vi "DumbDash Send.vi"(9 "Robot IP":string, 10 "data string":string) -> ()   [LabVIEW 2015]
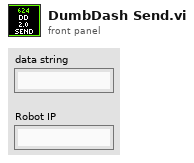
[diagram p1: front panel]
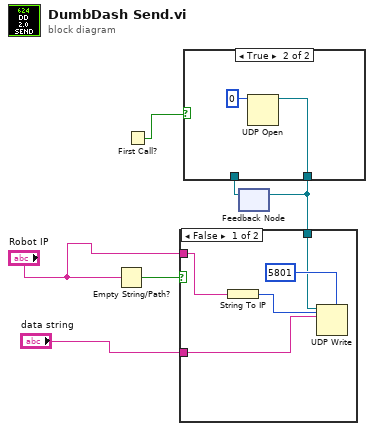
[diagram p0: block diagram]
diagram:
  n1 = Empty String/Path?(string/path="Robot IP") -> (empty?=w4:bool)
  n2 = First Call?() -> (First Call?: T/F=w3:bool)
  n3 = feedback #1() -> (w1:refnum<k16>)  [unwired: 1 in]
  n4 = case shown="True" w3 {
    tunnel: [w7 w9] -> w2
    tunnel: w1 -> [w7 _]
    frame False {
    }
    frame True {
      n5 = UDP Open(11:u16 0 ("port")) -> (port=w9:refnum<k16>)  [unwired: 4 in, 2 out]
    }
  }
  n6 = case shown="False" w4 {
    tunnel: "Robot IP" -> [w12 _]
    tunnel: "data string" -> [w11 _]
    tunnel: w2 -> [w10 _]
    frame False {
      n7 = String To IP(1:w12) -> (0:w13:u32)
      n8 = UDP Write(address=w13, port or service name=u16 5801, connection ID=w10, data in=w11) -> ()  [unwired: 2 in, 2 out]
    }
    frame True {
      # "The robot IP is not\nready yet, don't try\nto send data"
    }
  }
  n9 = feedback-in #1(w2) -> ()
